vi "testCorrectData.vi"() -> ()   [LabVIEW 2019, in "TestCaseTest.lvlib" / "Theory.lvlib"]
uses:
  Theory.lvlib
  TestCaseTestSupport/FakeTheory.vi
  TestCase/Theory/Theory.lvclass
  TestCaseTestSupport/TestCaseTestSupport.lvlib
  Assertion/Assertion.lvlib
panel:
  out "error out":errorcluster
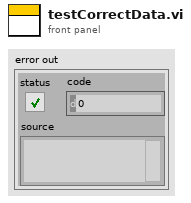
[diagram p1: front panel]
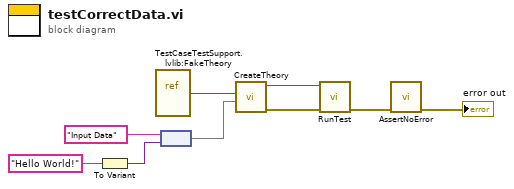
[diagram p0: block diagram]
diagram:
  n1 = To Variant(anything="Hello World!" ("key")) -> (Variant=w3:variant)
  n2 = vi-ref "TestCaseTestSupport.lvlib:FakeTheory.vi"() -> (w1:refnum<vi>)
  n3 = node("Input Data" ("key"), w3) -> (w4:map{string, variant})
  n4 = call "CreateTheory.vi"("Control Data"=w4, "VI Refnum"=w1) -> ("error out"=w8:errorcluster, "Theory"=w9:refnum<class "Theory.lvclass">)  [unwired: 8 in]
  n5 = call-dynamic "RunTest.vi"("error in (no error)"=w8, "Theory in"=w9) -> ("error out"=w7:errorcluster)  [unwired: 8 in, 1 out]
  n6 = call "AssertNoError.vi"("error in (no error)"=w7) -> ("error out"=→"error out":errorcluster)  [unwired: 10 in]
